vi "Untitled 22 (SubVI).vi"(9 "cpg":dbl, 10 "t4":dbl, 11 "t3t":dbl) -> (3 "wt":dbl)   [LabVIEW 2019]
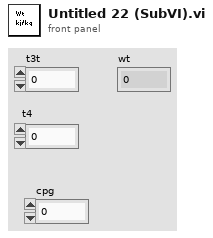
[diagram p1: front panel]
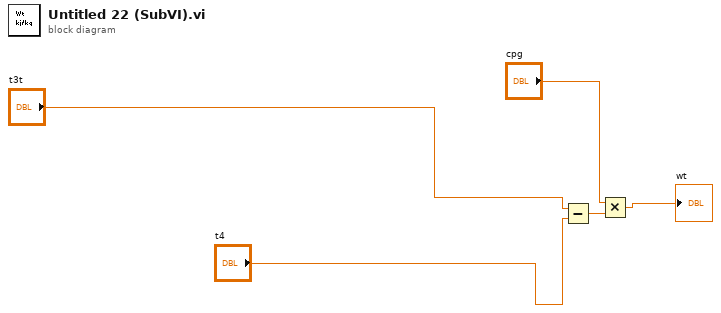
[diagram p0: block diagram]
diagram:
  n1 = Subtract(x="t3t", y="t4") -> (x-y=w4:dbl)
  n2 = Multiply(x="cpg", y=w4) -> (x*y=→"wt":dbl)
